vi "Math SubVI - Complex (SCR) (DBG OFF).vi"(1 "Input":dbl step=0.1 format="%.6f") -> (0 "Output":dbl format="%.6f")   [LabVIEW 2026]
doc: "This VI takes a floating-point number between 0 and 1 and maps it to another floating-point number between 0 and 1.\n\nEach repetition is a copy of the contents of \"Math SubVI - Medium (NR).vi\". By executing 10 repetitions, this VI should be roughly 10 times more computationally complex (10 times more CPU instructions) than the aforementioned subVI."
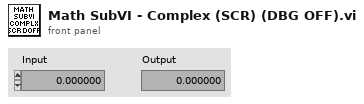
[diagram p1: front panel]
diagram:
  # "This VI takes a floating-point number between 0 and 1 and maps it to another floating-point number between 0 and 1.\n\nEach repetition is a copy of the contents of \"Math SubVI - Medium (NR).vi\". By executing 10 repetitions, this VI should be roughly 10 times more computationally complex (10 times more CPU instructions) than the aforementioned subVI."
  n1 = flat-sequence {
    tunnel: "Input" -> [w27]
    tunnel: [w13] -> w11
    frame #0 {
      # "Repetition 1."
      n2 = Square(x=w27) -> (x^2=w35:dbl)
      n3 = Multiply(x=w27, y=2.0 ("x")) -> (x*y=w32:dbl)
      n4 = Subtract(x=3.0, y=w32) -> (x-y=w31:dbl)
      n5 = Multiply(x=w35, y=w31) -> (x*y=w30:dbl)
      n6 = Multiply(x=6.283185307179586, y=w27) -> (x*y=w26:dbl)
      n7 = Sine(x=w26) -> (sin(x)=w25:dbl)
      n8 = Multiply(x=0.15, y=w25) -> (x*y=w24:dbl)
      n9 = Add(x=w30, y=w24) -> (x+y=w22:dbl)
      n10 = Subtract(x=w22, y=0.5 ("x")) -> (x-y=w21:dbl)
      n11 = Multiply(x=-6.0, y=w21) -> (x*y=w19:dbl)
      n12 = Exponential(1:w19) -> (0:w18:dbl)
      n13 = Increment(x=w18) -> (x+1=w17:dbl)
      n14 = Reciprocal(x=w17) -> (1/x=w16:dbl)
      n15 = In Range and Coerce(upper limit=1.0 ("x"), x=w16, lower limit=0.0 ("x")) -> (coerced(x)=w13:dbl)  [unwired: 1 out]
    }
  }
  n16 = flat-sequence {
    tunnel: w11 -> [w50]
    tunnel: [w36] -> w10
    frame #0 {
      # "Repetition 2"
      n17 = Square(x=w50) -> (x^2=w58:dbl)
      n18 = Multiply(x=w50, y=2.0 ("x")) -> (x*y=w55:dbl)
      n19 = Subtract(x=3.0, y=w55) -> (x-y=w54:dbl)
      n20 = Multiply(x=w58, y=w54) -> (x*y=w53:dbl)
      n21 = Multiply(x=6.283185307179586, y=w50) -> (x*y=w49:dbl)
      n22 = Sine(x=w49) -> (sin(x)=w48:dbl)
      n23 = Multiply(x=0.15, y=w48) -> (x*y=w47:dbl)
      n24 = Add(x=w53, y=w47) -> (x+y=w45:dbl)
      n25 = Subtract(x=w45, y=0.5 ("x")) -> (x-y=w44:dbl)
      n26 = Multiply(x=-6.0, y=w44) -> (x*y=w42:dbl)
      n27 = Exponential(1:w42) -> (0:w41:dbl)
      n28 = Increment(x=w41) -> (x+1=w40:dbl)
      n29 = Reciprocal(x=w40) -> (1/x=w39:dbl)
      n30 = In Range and Coerce(upper limit=1.0 ("x"), x=w39, lower limit=0.0 ("x")) -> (coerced(x)=w36:dbl)  [unwired: 1 out]
    }
  }
  n31 = flat-sequence {
    tunnel: w10 -> [w73]
    tunnel: [w59] -> w9
    frame #0 {
      # "Repetition 3"
      n32 = Square(x=w73) -> (x^2=w81:dbl)
      n33 = Multiply(x=w73, y=2.0 ("x")) -> (x*y=w78:dbl)
      n34 = Subtract(x=3.0, y=w78) -> (x-y=w77:dbl)
      n35 = Multiply(x=w81, y=w77) -> (x*y=w76:dbl)
      n36 = Multiply(x=6.283185307179586, y=w73) -> (x*y=w72:dbl)
      n37 = Sine(x=w72) -> (sin(x)=w71:dbl)
      n38 = Multiply(x=0.15, y=w71) -> (x*y=w70:dbl)
      n39 = Add(x=w76, y=w70) -> (x+y=w68:dbl)
      n40 = Subtract(x=w68, y=0.5 ("x")) -> (x-y=w67:dbl)
      n41 = Multiply(x=-6.0, y=w67) -> (x*y=w65:dbl)
      n42 = Exponential(1:w65) -> (0:w64:dbl)
      n43 = Increment(x=w64) -> (x+1=w63:dbl)
      n44 = Reciprocal(x=w63) -> (1/x=w62:dbl)
      n45 = In Range and Coerce(upper limit=1.0 ("x"), x=w62, lower limit=0.0 ("x")) -> (coerced(x)=w59:dbl)  [unwired: 1 out]
    }
  }
  n46 = flat-sequence {
    tunnel: w9 -> [w96]
    tunnel: [w82] -> w8
    frame #0 {
      # "Repetition 4"
      n47 = Square(x=w96) -> (x^2=w104:dbl)
      n48 = Multiply(x=w96, y=2.0 ("x")) -> (x*y=w101:dbl)
      n49 = Subtract(x=3.0, y=w101) -> (x-y=w100:dbl)
      n50 = Multiply(x=w104, y=w100) -> (x*y=w99:dbl)
      n51 = Multiply(x=6.283185307179586, y=w96) -> (x*y=w95:dbl)
      n52 = Sine(x=w95) -> (sin(x)=w94:dbl)
      n53 = Multiply(x=0.15, y=w94) -> (x*y=w93:dbl)
      n54 = Add(x=w99, y=w93) -> (x+y=w91:dbl)
      n55 = Subtract(x=w91, y=0.5 ("x")) -> (x-y=w90:dbl)
      n56 = Multiply(x=-6.0, y=w90) -> (x*y=w88:dbl)
      n57 = Exponential(1:w88) -> (0:w87:dbl)
      n58 = Increment(x=w87) -> (x+1=w86:dbl)
      n59 = Reciprocal(x=w86) -> (1/x=w85:dbl)
      n60 = In Range and Coerce(upper limit=1.0 ("x"), x=w85, lower limit=0.0 ("x")) -> (coerced(x)=w82:dbl)  [unwired: 1 out]
    }
  }
  n61 = flat-sequence {
    tunnel: w8 -> [w119]
    tunnel: [w105] -> w7
    frame #0 {
      # "Repetition 5"
      n62 = Square(x=w119) -> (x^2=w127:dbl)
      n63 = Multiply(x=w119, y=2.0 ("x")) -> (x*y=w124:dbl)
      n64 = Subtract(x=3.0, y=w124) -> (x-y=w123:dbl)
      n65 = Multiply(x=w127, y=w123) -> (x*y=w122:dbl)
      n66 = Multiply(x=6.283185307179586, y=w119) -> (x*y=w118:dbl)
      n67 = Sine(x=w118) -> (sin(x)=w117:dbl)
      n68 = Multiply(x=0.15, y=w117) -> (x*y=w116:dbl)
      n69 = Add(x=w122, y=w116) -> (x+y=w114:dbl)
      n70 = Subtract(x=w114, y=0.5 ("x")) -> (x-y=w113:dbl)
      n71 = Multiply(x=-6.0, y=w113) -> (x*y=w111:dbl)
      n72 = Exponential(1:w111) -> (0:w110:dbl)
      n73 = Increment(x=w110) -> (x+1=w109:dbl)
      n74 = Reciprocal(x=w109) -> (1/x=w108:dbl)
      n75 = In Range and Coerce(upper limit=1.0 ("x"), x=w108, lower limit=0.0 ("x")) -> (coerced(x)=w105:dbl)  [unwired: 1 out]
    }
  }
  n76 = flat-sequence {
    tunnel: w7 -> [w142]
    tunnel: [w128] -> w6
    frame #0 {
      # "Repetition 6"
      n77 = Square(x=w142) -> (x^2=w150:dbl)
      n78 = Multiply(x=w142, y=2.0 ("x")) -> (x*y=w147:dbl)
      n79 = Subtract(x=3.0, y=w147) -> (x-y=w146:dbl)
      n80 = Multiply(x=w150, y=w146) -> (x*y=w145:dbl)
      n81 = Multiply(x=6.283185307179586, y=w142) -> (x*y=w141:dbl)
      n82 = Sine(x=w141) -> (sin(x)=w140:dbl)
      n83 = Multiply(x=0.15, y=w140) -> (x*y=w139:dbl)
      n84 = Add(x=w145, y=w139) -> (x+y=w137:dbl)
      n85 = Subtract(x=w137, y=0.5 ("x")) -> (x-y=w136:dbl)
      n86 = Multiply(x=-6.0, y=w136) -> (x*y=w134:dbl)
      n87 = Exponential(1:w134) -> (0:w133:dbl)
      n88 = Increment(x=w133) -> (x+1=w132:dbl)
      n89 = Reciprocal(x=w132) -> (1/x=w131:dbl)
      n90 = In Range and Coerce(upper limit=1.0 ("x"), x=w131, lower limit=0.0 ("x")) -> (coerced(x)=w128:dbl)  [unwired: 1 out]
    }
  }
  n91 = flat-sequence {
    tunnel: w6 -> [w165]
    tunnel: [w151] -> w5
    frame #0 {
      # "Repetition 7"
      n92 = Square(x=w165) -> (x^2=w173:dbl)
      n93 = Multiply(x=w165, y=2.0 ("x")) -> (x*y=w170:dbl)
      n94 = Subtract(x=3.0, y=w170) -> (x-y=w169:dbl)
      n95 = Multiply(x=w173, y=w169) -> (x*y=w168:dbl)
      n96 = Multiply(x=6.283185307179586, y=w165) -> (x*y=w164:dbl)
      n97 = Sine(x=w164) -> (sin(x)=w163:dbl)
      n98 = Multiply(x=0.15, y=w163) -> (x*y=w162:dbl)
      n99 = Add(x=w168, y=w162) -> (x+y=w160:dbl)
      n100 = Subtract(x=w160, y=0.5 ("x")) -> (x-y=w159:dbl)
      n101 = Multiply(x=-6.0, y=w159) -> (x*y=w157:dbl)
      n102 = Exponential(1:w157) -> (0:w156:dbl)
      n103 = Increment(x=w156) -> (x+1=w155:dbl)
      n104 = Reciprocal(x=w155) -> (1/x=w154:dbl)
      n105 = In Range and Coerce(upper limit=1.0 ("x"), x=w154, lower limit=0.0 ("x")) -> (coerced(x)=w151:dbl)  [unwired: 1 out]
    }
  }
  n106 = flat-sequence {
    tunnel: w5 -> [w188]
    tunnel: [w174] -> w4
    frame #0 {
      # "Repetition 7"
      n107 = Square(x=w188) -> (x^2=w196:dbl)
      n108 = Multiply(x=w188, y=2.0 ("x")) -> (x*y=w193:dbl)
      n109 = Subtract(x=3.0, y=w193) -> (x-y=w192:dbl)
      n110 = Multiply(x=w196, y=w192) -> (x*y=w191:dbl)
      n111 = Multiply(x=6.283185307179586, y=w188) -> (x*y=w187:dbl)
      n112 = Sine(x=w187) -> (sin(x)=w186:dbl)
      n113 = Multiply(x=0.15, y=w186) -> (x*y=w185:dbl)
      n114 = Add(x=w191, y=w185) -> (x+y=w183:dbl)
      n115 = Subtract(x=w183, y=0.5 ("x")) -> (x-y=w182:dbl)
      n116 = Multiply(x=-6.0, y=w182) -> (x*y=w180:dbl)
      n117 = Exponential(1:w180) -> (0:w179:dbl)
      n118 = Increment(x=w179) -> (x+1=w178:dbl)
      n119 = Reciprocal(x=w178) -> (1/x=w177:dbl)
      n120 = In Range and Coerce(upper limit=1.0 ("x"), x=w177, lower limit=0.0 ("x")) -> (coerced(x)=w174:dbl)  [unwired: 1 out]
    }
  }
  n121 = flat-sequence {
    tunnel: w4 -> [w211]
    tunnel: [w197] -> w3
    frame #0 {
      # "Repetition 8"
      n122 = Square(x=w211) -> (x^2=w219:dbl)
      n123 = Multiply(x=w211, y=2.0 ("x")) -> (x*y=w216:dbl)
      n124 = Subtract(x=3.0, y=w216) -> (x-y=w215:dbl)
      n125 = Multiply(x=w219, y=w215) -> (x*y=w214:dbl)
      n126 = Multiply(x=6.283185307179586, y=w211) -> (x*y=w210:dbl)
      n127 = Sine(x=w210) -> (sin(x)=w209:dbl)
      n128 = Multiply(x=0.15, y=w209) -> (x*y=w208:dbl)
      n129 = Add(x=w214, y=w208) -> (x+y=w206:dbl)
      n130 = Subtract(x=w206, y=0.5 ("x")) -> (x-y=w205:dbl)
      n131 = Multiply(x=-6.0, y=w205) -> (x*y=w203:dbl)
      n132 = Exponential(1:w203) -> (0:w202:dbl)
      n133 = Increment(x=w202) -> (x+1=w201:dbl)
      n134 = Reciprocal(x=w201) -> (1/x=w200:dbl)
      n135 = In Range and Coerce(upper limit=1.0 ("x"), x=w200, lower limit=0.0 ("x")) -> (coerced(x)=w197:dbl)  [unwired: 1 out]
    }
  }
  n136 = flat-sequence {
    tunnel: w3 -> [w234]
    tunnel: [w220] -> w2
    frame #0 {
      # "Repetition 9"
      n137 = Square(x=w234) -> (x^2=w242:dbl)
      n138 = Multiply(x=w234, y=2.0 ("x")) -> (x*y=w239:dbl)
      n139 = Subtract(x=3.0, y=w239) -> (x-y=w238:dbl)
      n140 = Multiply(x=w242, y=w238) -> (x*y=w237:dbl)
      n141 = Multiply(x=6.283185307179586, y=w234) -> (x*y=w233:dbl)
      n142 = Sine(x=w233) -> (sin(x)=w232:dbl)
      n143 = Multiply(x=0.15, y=w232) -> (x*y=w231:dbl)
      n144 = Add(x=w237, y=w231) -> (x+y=w229:dbl)
      n145 = Subtract(x=w229, y=0.5 ("x")) -> (x-y=w228:dbl)
      n146 = Multiply(x=-6.0, y=w228) -> (x*y=w226:dbl)
      n147 = Exponential(1:w226) -> (0:w225:dbl)
      n148 = Increment(x=w225) -> (x+1=w224:dbl)
      n149 = Reciprocal(x=w224) -> (1/x=w223:dbl)
      n150 = In Range and Coerce(upper limit=1.0 ("x"), x=w223, lower limit=0.0 ("x")) -> (coerced(x)=w220:dbl)  [unwired: 1 out]
    }
  }
  n151 = flat-sequence {
    tunnel: w2 -> [w257]
    tunnel: [w243] -> w1
    frame #0 {
      # "Repetition 10"
      n152 = Square(x=w257) -> (x^2=w265:dbl)
      n153 = Multiply(x=w257, y=2.0 ("x")) -> (x*y=w262:dbl)
      n154 = Subtract(x=3.0, y=w262) -> (x-y=w261:dbl)
      n155 = Multiply(x=w265, y=w261) -> (x*y=w260:dbl)
      n156 = Multiply(x=6.283185307179586, y=w257) -> (x*y=w256:dbl)
      n157 = Sine(x=w256) -> (sin(x)=w255:dbl)
      n158 = Multiply(x=0.15, y=w255) -> (x*y=w254:dbl)
      n159 = Add(x=w260, y=w254) -> (x+y=w252:dbl)
      n160 = Subtract(x=w252, y=0.5 ("x")) -> (x-y=w251:dbl)
      n161 = Multiply(x=-6.0, y=w251) -> (x*y=w249:dbl)
      n162 = Exponential(1:w249) -> (0:w248:dbl)
      n163 = Increment(x=w248) -> (x+1=w247:dbl)
      n164 = Reciprocal(x=w247) -> (1/x=w246:dbl)
      n165 = In Range and Coerce(upper limit=1.0 ("x"), x=w246, lower limit=0.0 ("x")) -> (coerced(x)=w243:dbl)  [unwired: 1 out]
    }
  }
  "Output" <- w1
